vi "usb capture read.vi"(10 "read_data":u8[](array[numeric])=array[65536 elements], 11 "len":i32) -> (2 "read_data out":u8[](array[numeric]), 3 "function return":bool)   [LabVIEW 2018, in "Dll1_x64_191014_0.lvlib"]
doc: "__declspec(dllexport) bool usb_capture_read(int len, unsigned char read_data[65536]);"
uses:
  Dll1_x64_191014_0.lvlib
  Dll1.dll
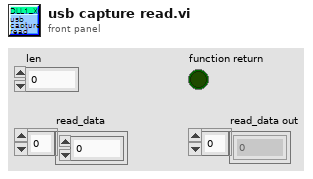
[diagram p1: front panel]
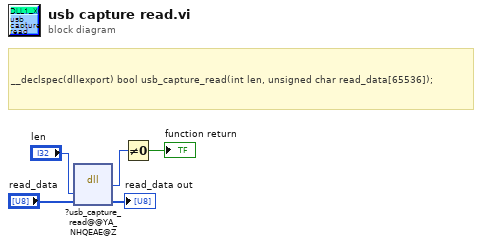
[diagram p0: block diagram]
diagram:
  # "__declspec(dllexport) bool usb_capture_read(int len, unsigned char read_data[65536]);"
  n1 = dll-call lib="PTH2zabs CUsersLenovoDesktopDHCC실험2#lux image capture_0.9.1.1_Temporaryuser.libDll1_x64_191014_0Dll1.*" fn="?usb_capture_read@@YA_NHQEAE@Z"("len"="len", "read_data"="read_data") -> (w4:u8, "read_data"=→"read_data out":u8[])  [unwired: 4 in, 2 out]
  n2 = Not Equal To 0?(x=w4) -> (x != 0?=→"function return":bool)
